vi "SetS0Bit.vi"(0 "drv":u32, 1 "Address":u8, 2 "bitnumber":u32) -> ()   [LabVIEW 2015]
uses:
  ESLSCDLL.dll
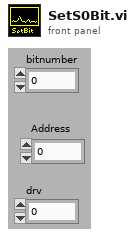
[diagram p1: front panel]
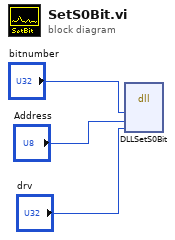
[diagram p0: block diagram]
diagram:
  n1 = dll-call lib="C:/ENTW/PCIE/64bit/lv64/lv15_act2018/board.vis/ESLSCDLL.dll" fn="DLLSetS0Bit" ("lwlscdll.dll:DLLRsTOREG")("bitnumber"="bitnumber", "Address"="Address", "drv"="drv") -> ()  [unwired: 7 in, 2 out]
